vi "Rambo Code 2.vi"(0 "Color Mode (Color Threshold 1)":u16(ring)=1 items=["RGB", "HSL", "HSV", "HSI"], 1 "Red or Hue Range (Color Threshold 1)":cluster{"Lower value":i32, "Upper value":i32}={"Lower value"=52, "Upper value"=124}, 2 "Green or Sat Range (Color Threshold 1)":cluster{"Lower value":i32, "Upper value":i32}={"Lower value"=171, "Upper value"=255}, 3 "Blue or Luma or Val or Inten Range (Color Threshold 1)":cluster{"Lower value":i32, "Upper value":i32}={"Lower value"=136, "Upper value"=255}, 4 "Image In":T1(plugin-control)) -> (20 "Rectangles (Shape Detection 1)":T2(array[cluster]) {"Corners"."Y" format="%.2f"; "Corners"."X" format="%.2f"}, 21 "Number of Particles (Particle Analysis 1)":i32, 22 "Particle Measurements (Pixels) (Particle Analysis 1)":dbl[][](array[numeric]) format="%.2f", 24 "Image Out":T1(plugin-control), 27 "error out":errorcluster)   [LabVIEW 2012]
uses:
  <vilib>/vision/NI_Vision_Development_Module.lvlib
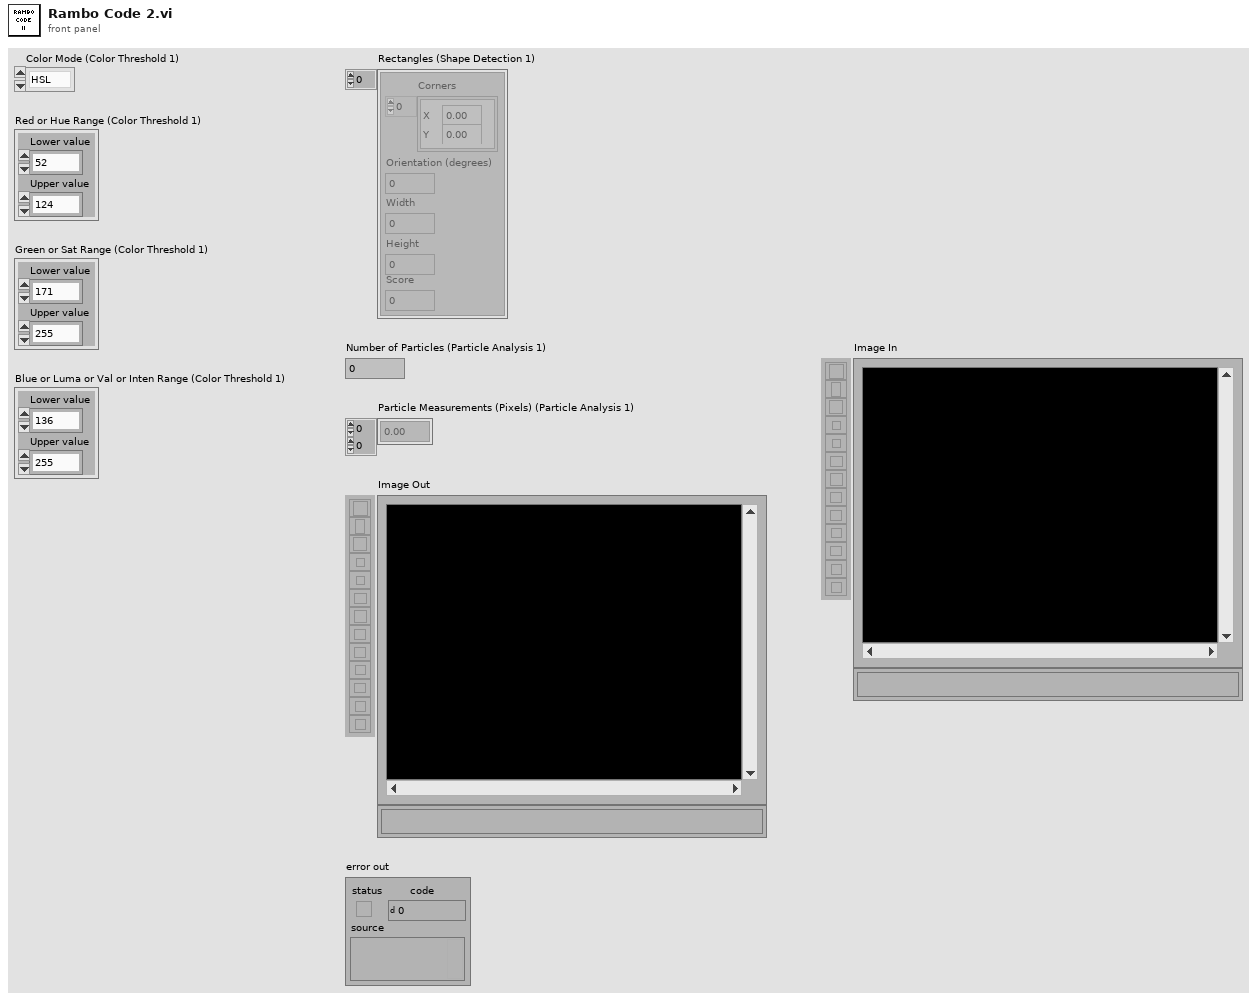
[diagram p1: front panel]
types:
  T1 = typedef "IMAQ Image.ctl" = refnum<image>
  T2 = cluster{"Corners":cluster{"X":sgl, "Y":sgl}[], "Orientation (degrees)":dbl, "Width":dbl, "Height":dbl, "Score":dbl}[]
  T3 = cluster{"Min Major Radius":dbl, "Max Major Radius":dbl, "Min Minor Radius":dbl, "Max Minor Radius":dbl}
  T4 = cluster{"Extraction Mode":u32, "Edge Threshold":i32, "Edge Filter Size":u32, "Min Length":i32, "Row Search Step Size":i32, "Col Search Step Size":i32, "Max Endpoint Gap":i32, "Closed":bool, "Subpixel":bool}
  T5 = cluster{"Rotation":bool, "Scale":bool, "Occlusion":bool, "Range Settings":cluster{"Match Constraints":u32, "Min":dbl, "Max":dbl}[]}
  T6 = cluster{"Global Rectangle":i32[], "Contours":cluster{"ID":enum32{"External", "Internal"}, "Type":u32, "Coordinates":i32[]}[]}
  T7 = enum32{"AutoM", "Close", "Dilate", "Erode", "Gradient", "Gradient out", "Gradient in", "Hit miss", "Open", "PClose", "POpen", "Thick", "Thin"}
  T8 = cluster{"histogram":u32[], "Minimal Value":sgl, "Maximal Value":sgl, "Starting Value":sgl, "Interval Width":sgl, "Mean Value":sgl, "Standard  Variation":sgl, "Area (pixels)":i32}
  T9 = typedef "Image Type" = u32
  T10 = cluster{"Corners":cluster{"X":sgl, "Y":sgl}[], "Angle":dbl, "Width":dbl, "Height":dbl, "Score":dbl}[]
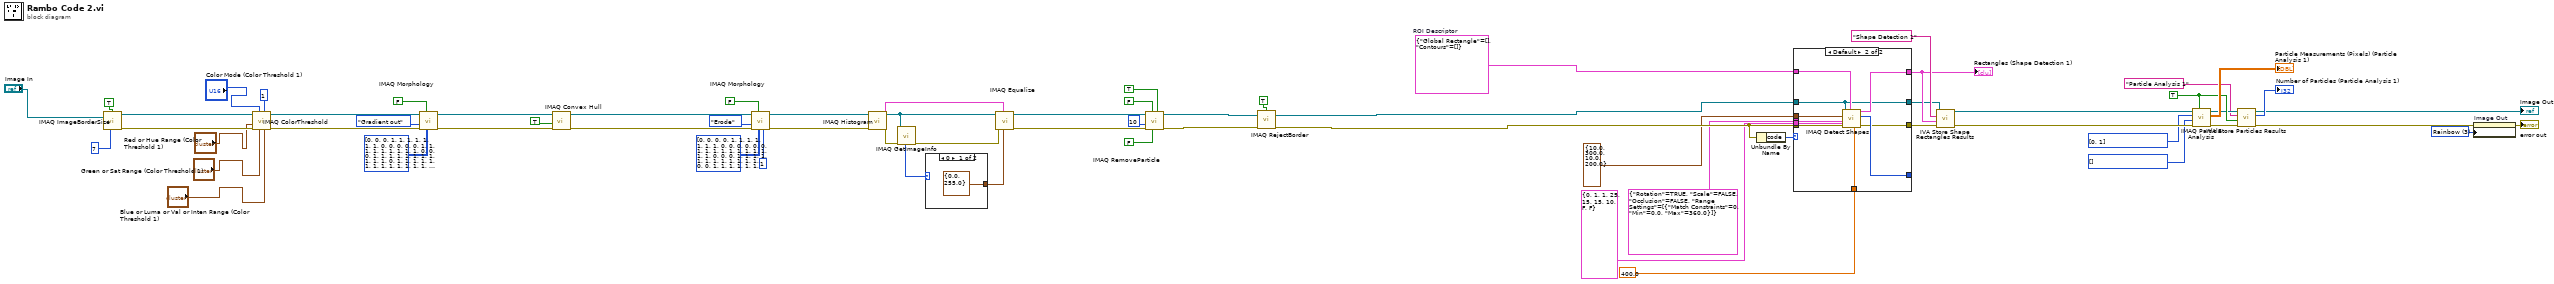
[diagram p0: block diagram]
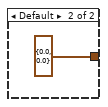
[diagram p3: hidden frame]
diagram:
  w3 = u32 3 items=["Grayscale", "Binary", "Gradient", "Rainbow", "Temperature", "User Defined"] ("Palette")
  w13 = i32[] [] items=["Center of Mass X", "Center of Mass Y", "First Pixel X", "First Pixel Y", "Bounding Rect Left", "Bounding Rect Top", "Bounding Rect Right", "Bounding Rect Bottom", "Max Feret Diameter Start X", "Max Feret Diameter Start Y", "Max Feret Diameter End X", "Max Feret Diameter End Y", "Max Horiz. Segment Length Left", "Max Horiz. Segment Length Right", "Max Horiz. Segment Length Row", "-", "Bounding Rect Width", "Bounding Rect Height", "Bounding Rect Diagonal", "Perimeter", "Convex Hull Perimeter", "Holes' Perimeter", "Max Feret Diameter", "Equivalent Ellipse Major Axis", "Equivalent Ellipse Minor Axis", "Equivalent Ellipse Minor Axis (Feret)", "Equivalent Rect Long Side", "Equivalent Rect Short Side", "Equivalent Rect Diagonal", "Equivalent Rect Short Side (Feret)", "Average Horiz. Segment Length", "Average Vert. Segment Length", "Hydraulic Radius", "Waddel Disk Diameter", "-", "Area", "Holes' Area", "Particle & Holes' Area", "Convex Hull Area", "Image Area", "-", "Number of Holes", "Number of Horiz. Segments", "Number of Vert. Segments", "-", "Orientation", "Max Feret Diameter Orientation", "-", "% Area/Image Area", "% Area/(Particle & Holes' Area)", "Ratio of Equivalent Ellipse Axes", "Ratio of Equivalent Rect Sides", "-", "Elongation Factor", "Compactness Factor", "Heywood Circularity Factor", "Type Factor", "-", "Sum X", "Sum Y", "Sum XX", "Sum XY", "Sum YY", "Sum XXX", "Sum XXY", "Sum XYY", "Sum YYY", "-", "Moment of Inertia XX", "Moment of Inertia XY", "Moment of Inertia YY", "Moment of Inertia XXX", "Moment of Inertia XXY", "Moment of Inertia XYY", "Moment of Inertia YYY", "Norm. Moment of Inertia XX", "Norm. Moment of Inertia XY", "Norm. Moment of Inertia YY", "Norm. Moment of Inertia XXX", "Norm. Moment of Inertia XXY", "Norm. Moment of Inertia XYY", "Norm. Moment of Inertia YYY", "Hu Moment 1", "Hu Moment 2", "Hu Moment 3", "Hu Moment 4", "Hu Moment 5", "Hu Moment 6", "Hu Moment 7"] ("Real-World Measurements")
  w14 = i32[] [0, 1] items=["Center of Mass X", "Center of Mass Y", "First Pixel X", "First Pixel Y", "Bounding Rect Left", "Bounding Rect Top", "Bounding Rect Right", "Bounding Rect Bottom", "Max Feret Diameter Start X", "Max Feret Diameter Start Y", "Max Feret Diameter End X", "Max Feret Diameter End Y", "Max Horiz. Segment Length Left", "Max Horiz. Segment Length Right", "Max Horiz. Segment Length Row", "-", "Bounding Rect Width", "Bounding Rect Height", "Bounding Rect Diagonal", "Perimeter", "Convex Hull Perimeter", "Holes' Perimeter", "Max Feret Diameter", "Equivalent Ellipse Major Axis", "Equivalent Ellipse Minor Axis", "Equivalent Ellipse Minor Axis (Feret)", "Equivalent Rect Long Side", "Equivalent Rect Short Side", "Equivalent Rect Diagonal", "Equivalent Rect Short Side (Feret)", "Average Horiz. Segment Length", "Average Vert. Segment Length", "Hydraulic Radius", "Waddel Disk Diameter", "-", "Area", "Holes' Area", "Particle & Holes' Area", "Convex Hull Area", "Image Area", "-", "Number of Holes", "Number of Horiz. Segments", "Number of Vert. Segments", "-", "Orientation", "Max Feret Diameter Orientation", "-", "% Area/Image Area", "% Area/(Particle & Holes' Area)", "Ratio of Equivalent Ellipse Axes", "Ratio of Equivalent Rect Sides", "-", "Elongation Factor", "Compactness Factor", "Heywood Circularity Factor", "Type Factor", "-", "Sum X", "Sum Y", "Sum XX", "Sum XY", "Sum YY", "Sum XXX", "Sum XXY", "Sum XYY", "Sum YYY", "-", "Moment of Inertia XX", "Moment of Inertia XY", "Moment of Inertia YY", "Moment of Inertia XXX", "Moment of Inertia XXY", "Moment of Inertia XYY", "Moment of Inertia YYY", "Norm. Moment of Inertia XX", "Norm. Moment of Inertia XY", "Norm. Moment of Inertia YY", "Norm. Moment of Inertia XXX", "Norm. Moment of Inertia XXY", "Norm. Moment of Inertia XYY", "Norm. Moment of Inertia YYY", "Hu Moment 1", "Hu Moment 2", "Hu Moment 3", "Hu Moment 4", "Hu Moment 5", "Hu Moment 6", "Hu Moment 7"] ("Pixel Measurements")
  w10 = TRUE ("Connectivity 4/8 (8)")
  w22 = T6 {"Global Rectangle"=[], "Contours"=[]}  # ROI Descriptor
  n1 = call "IMAQ ImageBorderSize"("Get/Set Status? (Set)"=TRUE, "Image"="Image In", "Image border size in"=7 ("Border Size")) -> ("Image Out"=w58:T1, "error out"=w66:errorcluster)  [unwired: 1 in, 1 out]
  n2 = call "IMAQ ColorThreshold"("Blue or Luma or Val or Inten Range"="Blue or Luma or Val or Inten Range (Color Threshold 1)", "Replace Value"=1, "Green or Sat Range"="Green or Sat Range (Color Threshold 1)", "Color Mode"="Color Mode (Color Threshold 1)", "error in (no error)"=w66, "Red or Hue Range"="Red or Hue Range (Color Threshold 1)", "Image Src"=w58) -> ("error out"=w57:errorcluster, "Image Dst Out"=w53:T1)  [unwired: 1 in, 2 out]
  n3 = call "IMAQ Morphology"("Structuring Element"=i32[][] [[0, 0, 0, 1, 1, 1, 1, 1, 1, 1, 0, 0, 0], [0, 0, 1, 1, 1, 1, 1, 1, 1, 1, 1, 0, 0], [0, 1, 1, 1, 1, 1, 1, 1, 1, 1, 1, 1, 0], [1, 1, 1, 1, 1, 1, 1, 1, 1, 1, 1, 1, 1], [1, 1, 1, 1, 1, 1, 1, 1, 1, 1, 1, 1, 1], [1, 1, 1, 1, 1, 1, 1, 1, 1, 1, 1, 1, 1], [1, 1, 1, 1, 1, 1, 1, 1, 1, 1, 1, 1, 1], [1, 1, 1, 1, 1, 1, 1, 1, 1, 1, 1, 1, 1], [1, 1, 1, 1, 1, 1, 1, 1, 1, 1, 1, 1, 1], [1, 1, 1, 1, 1, 1, 1, 1, 1, 1, 1, 1, 1], [0, 1, 1, 1, 1, 1, 1, 1, 1, 1, 1, 1, 0], [0, 0, 1, 1, 1, 1, 1, 1, 1, 1, 1, 0, 0], [0, 0, 0, 1, 1, 1, 1, 1, 1, 1, 0, 0, 0]], "Square/Hexa (Square)"=FALSE, "error in (no error)"=w57, "Operation"=T7."Gradient out", "Image Src"=w53) -> ("error out"=w52:errorcluster, "Image Dst Out"=w51:T1)  [unwired: 2 in, 3 out]
  n4 = call "IMAQ Convex Hull"("error in (no error)"=w52, "Connectivity 4/8 (8)"=TRUE, "Image Src"=w51) -> ("error out"=w49:errorcluster, "Image Dst Out"=w44:T1)  [unwired: 1 in, 6 out]
  n5 = call "IMAQ Morphology"("Number of iterations (1)"=1, "Structuring Element"=i32[][] [[0, 0, 0, 0, 1, 1, 1, 1, 1, 1, 1, 0, 0, 0, 0], [0, 0, 1, 1, 1, 1, 1, 1, 1, 1, 1, 1, 1, 0, 0], [0, 1, 1, 1, 1, 1, 1, 1, 1, 1, 1, 1, 1, 1, 0], [0, 1, 1, 1, 1, 1, 1, 1, 1, 1, 1, 1, 1, 1, 0], [1, 1, 1, 1, 1, 1, 1, 1, 1, 1, 1, 1, 1, 1, 1], [1, 1, 1, 1, 1, 1, 1, 1, 1, 1, 1, 1, 1, 1, 1], [1, 1, 1, 1, 1, 1, 1, 1, 1, 1, 1, 1, 1, 1, 1], [1, 1, 1, 1, 1, 1, 1, 1, 1, 1, 1, 1, 1, 1, 1], [1, 1, 1, 1, 1, 1, 1, 1, 1, 1, 1, 1, 1, 1, 1], [1, 1, 1, 1, 1, 1, 1, 1, 1, 1, 1, 1, 1, 1, 1], [1, 1, 1, 1, 1, 1, 1, 1, 1, 1, 1, 1, 1, 1, 1], [0, 1, 1, 1, 1, 1, 1, 1, 1, 1, 1, 1, 1, 1, 0], [0, 1, 1, 1, 1, 1, 1, 1, 1, 1, 1, 1, 1, 1, 0], [0, 0, 1, 1, 1, 1, 1, 1, 1, 1, 1, 1, 1, 0, 0], [0, 0, 0, 0, 1, 1, 1, 1, 1, 1, 1, 0, 0, 0, 0]], "Square/Hexa (Square)"=FALSE, "error in (no error)"=w49, "Operation"=T7."Erode", "Image Src"=w44) -> ("error out"=w43:errorcluster, "Image Dst Out"=w39:T1)  [unwired: 1 in, 3 out]
  n6 = call "IMAQ Histogram"("error in (no error)"=w43, "Image"=w39) -> ("error out"=w38:errorcluster, "Histogram Report"=w41:T8)  [unwired: 3 in, 5 out]
  n7 = call "IMAQ GetImageInfo"("error in (no error)"=w38, "Image"=w39) -> ("error out"=w37:errorcluster, "Image Type"=w40:T9)  [unwired: 8 out]
  n8 = case shown="0" w40 {
    tunnel: [cluster{"Minimum":sgl, "Maximum":sgl} {"Minimum"=0.0, "Maximum"=255.0} ("Range") cluster{"Minimum":sgl, "Maximum":sgl} {"Minimum"=0.0, "Maximum"=0.0} ("Range")] -> w36
    frame 0 {
    }
    frame Default {
    }
  }
  n9 = call "IMAQ Equalize"("Range"=w36, "Histogram Report"=w41, "error in (no error)"=w37, "Image Src"=w39) -> ("error out"=w42:errorcluster, "Image Dst Out"=w31:T1)  [unwired: 2 in, 4 out]
  n10 = call "IMAQ RemoveParticle"("Connectivity 4/8 (8)"=TRUE, "Low Pass/High Pass (Low)"=FALSE, "Square/Hexa (Square)"=FALSE, "error in (no error)"=w42, "Number of Erosion"=10, "Image Src"=w31) -> ("error out"=w30:errorcluster, "Image Dst Out"=w28:T1)  [unwired: 1 in, 3 out]
  n11 = call "IMAQ RejectBorder"("error in (no error)"=w30, "Image Src"=w28, "Connectivity 4/8 (8)"=TRUE) -> ("error out"=w27:errorcluster, "Image Dst Out"=w21:T1)  [unwired: 1 in, 2 out]
  n12 = Unbundle By Name(w27) -> ("code"=w15:i32)
  n13 = case shown="Default" w15 {
    tunnel: w27 -> [_ w79]
    tunnel: [_ w78] -> _
    tunnel: T5 {"Rotation"=TRUE, "Scale"=FALSE, "Occlusion"=FALSE, "Range Settings"=[{"Match Constraints"=0, "Min"=0.0, "Max"=360.0}]} ("Match Options") -> [_ w77]
    tunnel: T4 {"Extraction Mode"=0, "Edge Threshold"=1, "Edge Filter Size"=1, "Min Length"=25, "Row Search Step Size"=15, "Col Search Step Size"=15, "Max Endpoint Gap"=10, "Closed"=FALSE, "Subpixel"=FALSE} ("Curve Parameters") -> [_ w76]
    tunnel: 400.0 ("Minimum match score") -> [_ w75]
    tunnel: T3 {"Min Major Radius"=10.0, "Max Major Radius"=300.0, "Min Minor Radius"=10.0, "Max Minor Radius"=200.0} ("Rectangle Descriptor") -> [_ w74]
    tunnel: w22 -> [_ w73]
    tunnel: w21 -> [w69 w70]
    tunnel: [_ w72] -> w20
    tunnel: [_ w71] -> w17
    tunnel: [w69 w70] -> w16
    frame -1074396199, -1074396198 {
      # "Discard Coordinate System Error"
    }
    frame Default {
      n14 = call-poly "IMAQ Detect Shapes"("Minimum match score"=w75, "Curve Parameters"=w76, "ROI Descriptor"=w73, "error in (no error)"=w79, "Match Options"=w77, "Rectangle Descriptor"=w74, "Image"=w70) -> ("error out"=w72:errorcluster, "Number of Matches Returned"=w78:i32, "Rectangles"=w71:T10)  [unwired: 2 out]
    }
  }
  "Rectangles (Shape Detection 1)" <- w17
  n15 = call <vilib>:"IVA Store Shape Rectangles Results.vi"("error in (no error)"=w20, "Rectangles"=w17, "Step Name"="Shape Detection 1", "Image in"=w16) -> ("error out"=w19:errorcluster, "Image dup"=w11:T1)  [unwired: 6 out]
  n16 = call "IMAQ Particle Analysis"("Connectivity 4/8 (8)"=w10, "error in (no error)"=w19, "Real-World Measurements"=w13, "Pixel Measurements"=w14, "Image"=w11) -> ("error out"=w7:errorcluster, "Particle Measurements (Pixels)"=→"Particle Measurements (Pixels) (Particle Analysis 1)":dbl[][], "Image Out (duplicate)"=w9:T1)  [unwired: 4 out]
  n17 = call <vilib>:"IVA Store Particles Results.vi"("error in (no error)"=w7, "Connectivity 4/8 (8)"=w10, "Step Name"="Particle Analysis 1", "Image in"=w9) -> ("error out"=w6:errorcluster, "Number of Particles"=→"Number of Particles (Particle Analysis 1)":i32, "Image dup"=→"Image Out":T1)  [unwired: 5 out]
  n18 = property on="Image Out" class="ImageControl"(error in=w6, "Palette:Palette Type"=w3) -> (error out=→"error out":errorcluster)  [unwired: 1 in, 1 out]
